vi "MT Calculate BER After Trigger (Fibonacci PN Sequence).vi"(0 "input bit stream":i8[](array[numeric]), 5 "PN sequence order (9)":i32=9, 7 "BER trigger threshold (0.1)":dbl=0.1 format="%.4f", 9 "confidence (0.95)":dbl=0.95 format="%.4f", 11 "error in (no error)":errorcluster, 13 "reset? (T)":bool=TRUE) -> (4 "BER":dbl format="%.4f", 6 "accumulated BER":dbl format="%.4f", 8 "trigger found?":bool, 10 "trigger found index (bits)":u32, 15 "error out":errorcluster)   [LabVIEW 2020, in "niDMT.lvlib"]
doc: "This polymorphic instance calculates the average BER against a Fibonacci PN sequence. The sequence must be the same as the PN sequence generated by the Fibonacci instance of the MT Generate Bits (poly) VI with a matching PN order."
uses:
  <vilib>/addons/Modulation/niDMT.lvlib
  <vilib>/addons/Modulation/niAMT.lvlib
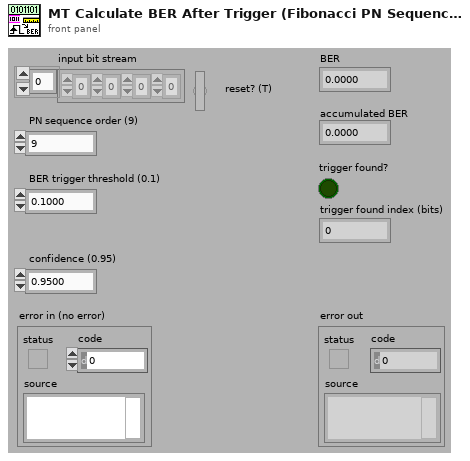
[diagram p1: front panel]
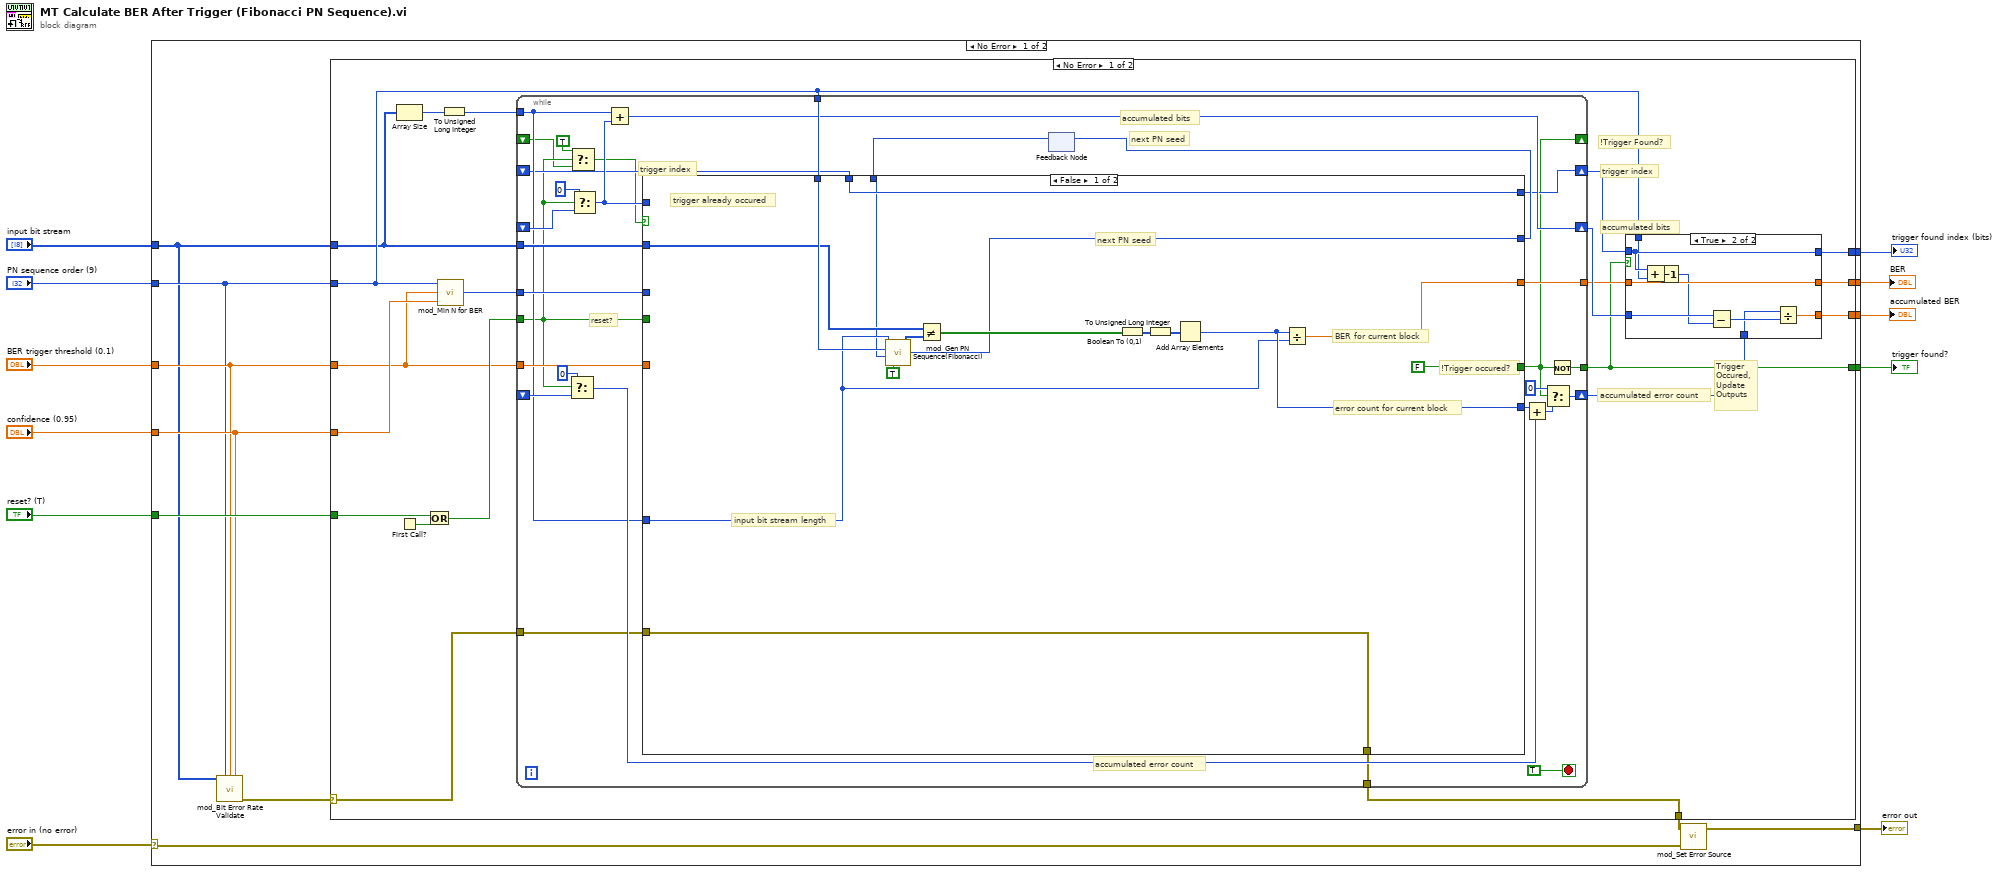
[diagram p0: block diagram]
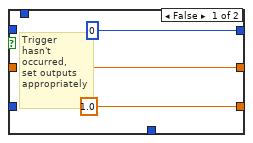
[diagram p2: hidden frame]
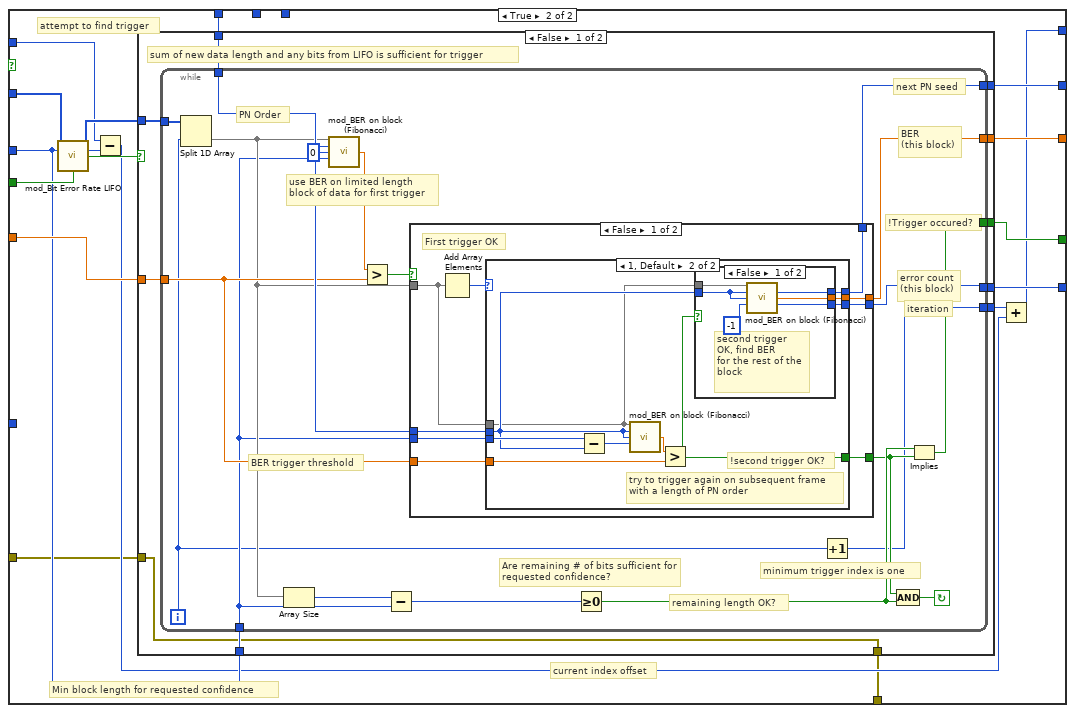
[diagram p3: hidden frame]
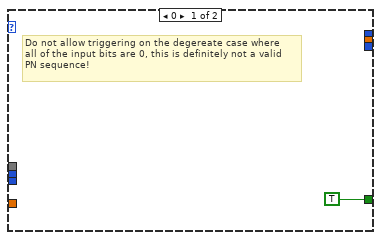
[diagram p4: hidden frame]
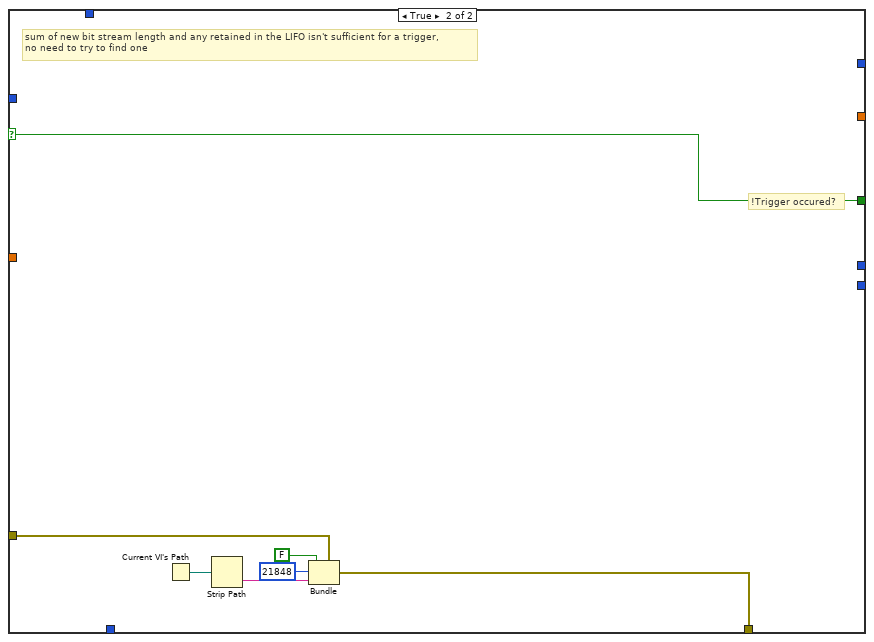
[diagram p7: hidden frame]
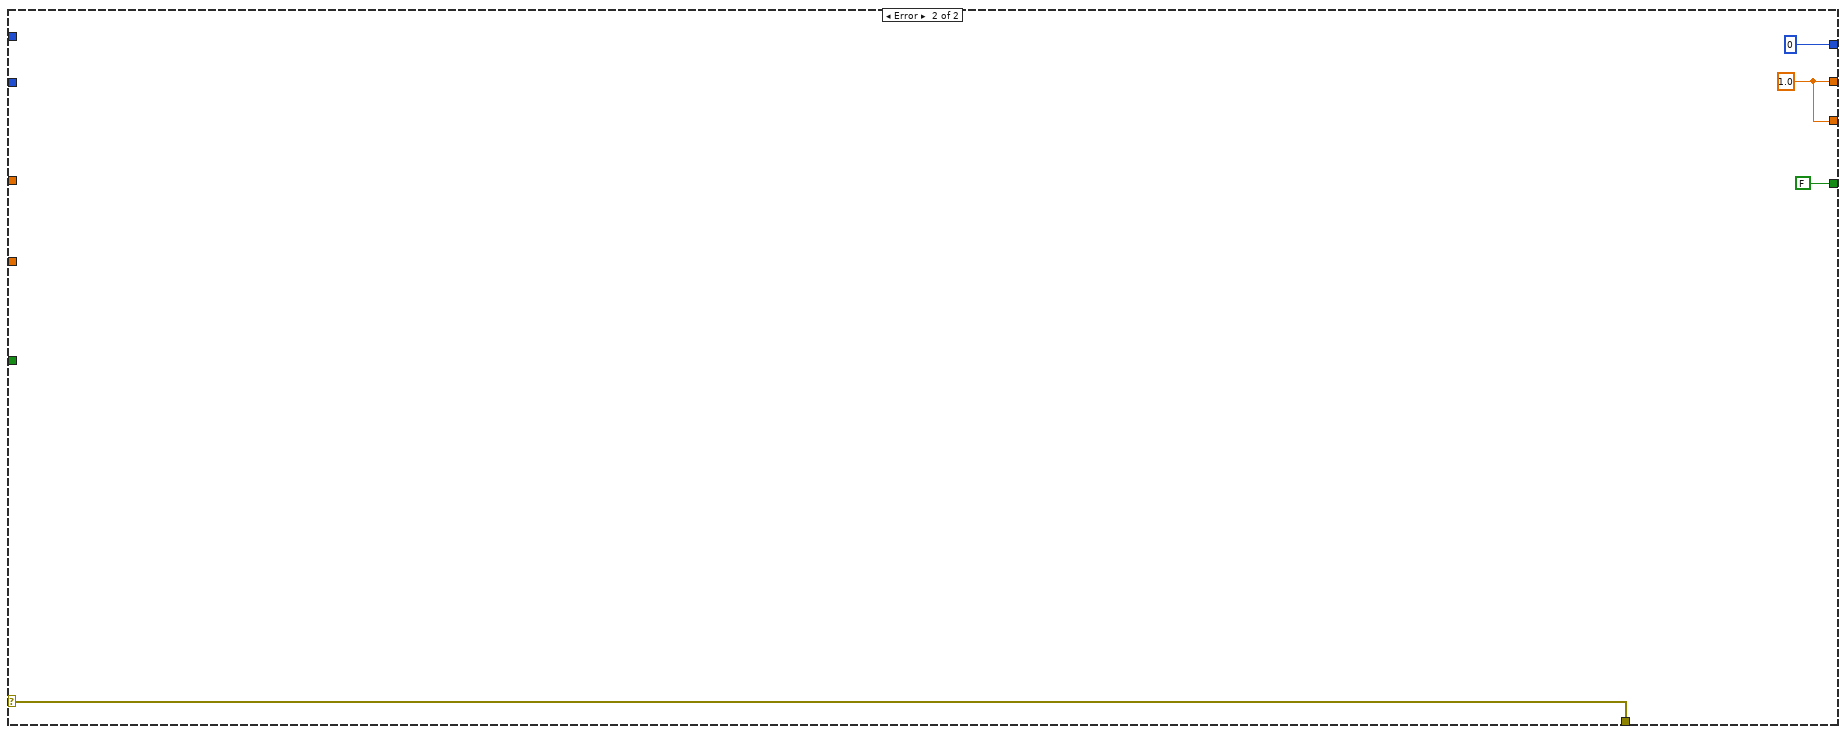
[diagram p8: hidden frame]
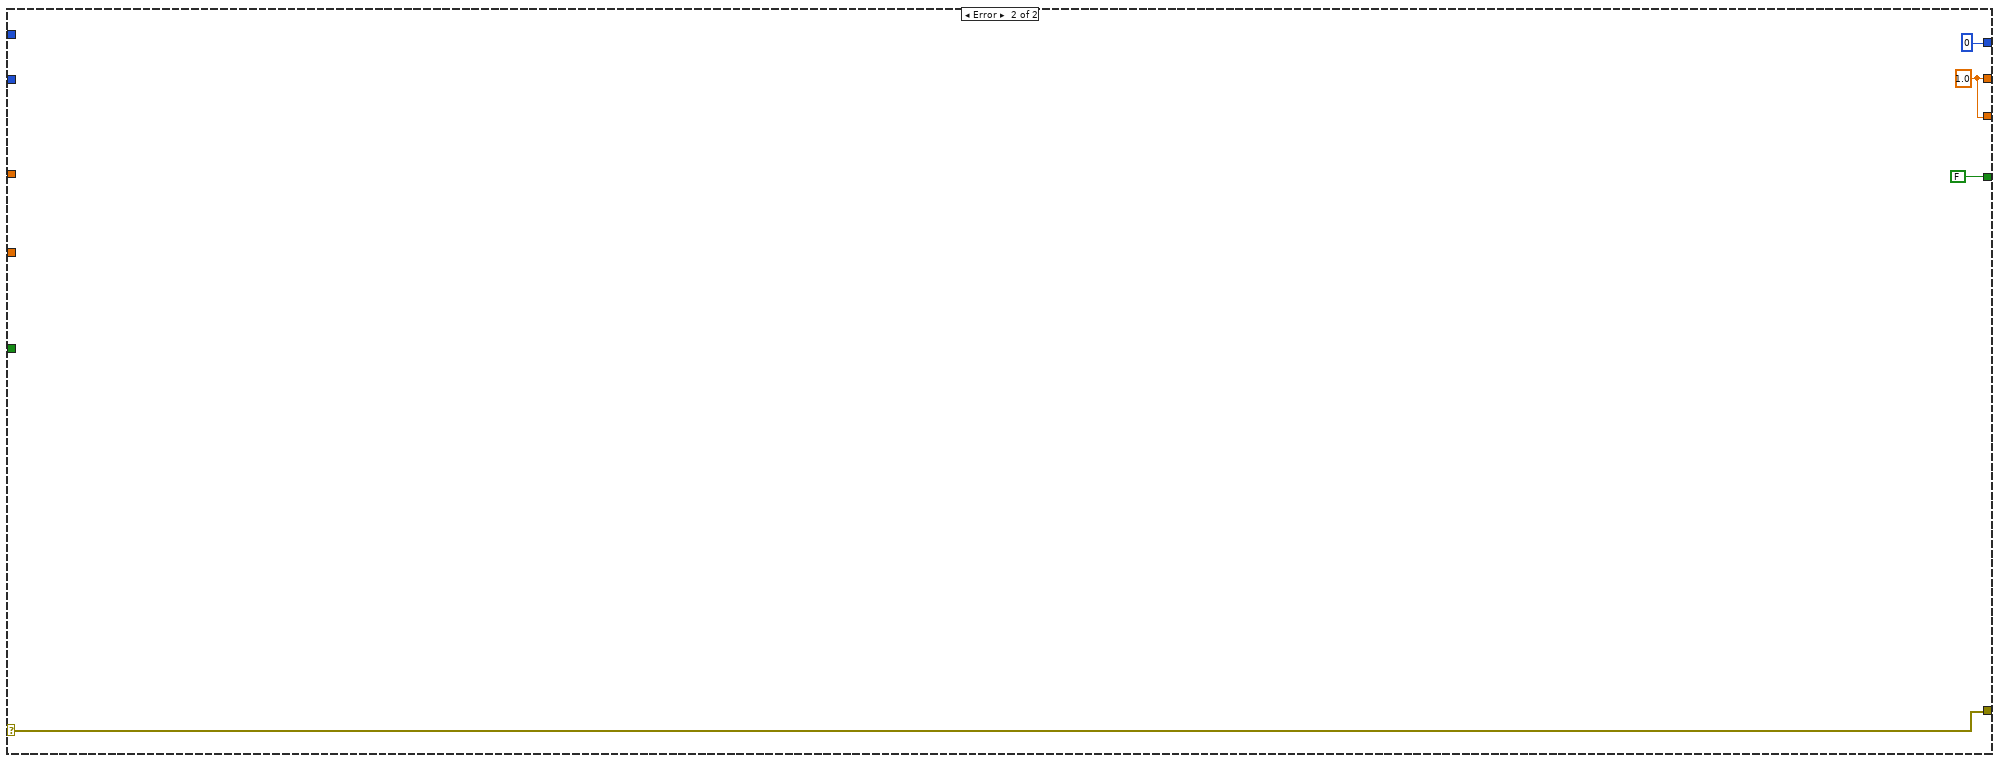
[diagram p9: hidden frame]
diagram:
  n1 = case shown="No Error" "error in (no error)" {
    selector: "error in (no error)" -> [w15 w189]
    tunnel: "reset? (T)" -> [w22 _]
    tunnel: "PN sequence order (9)" -> [w19 _]
    tunnel: "BER trigger threshold (0.1)" -> [w20 _]
    tunnel: "input bit stream" -> [w18 _]
    tunnel: [w24 w188] -> w8
    tunnel: "confidence (0.95)" -> [w21 _]
    tunnel: [w23 w189] -> w6
    tunnel: [w14 w188] -> w3
    tunnel: [w13 u32 0 ("t")] -> w2
    tunnel: [w12 FALSE] -> w1
    frame No Error {
      n2 = call <vilib>:"mod_Bit Error Rate Validate.vi"("Input Bit Stream"=w18, "PN Sequence Order (9)"=w19, "BER Sync Threshold (0.2)"=w20, "confidence (0.95)"=w21) -> ("error out"=w17:errorcluster)  [unwired: 1 in, 10 out]
      n3 = case shown="No Error" w17 {
        selector: w17 -> [w26 w185]
        tunnel: w19 -> [w30 _]
        tunnel: w20 -> [w31 _]
        tunnel: w18 -> [w28 _]
        tunnel: [w37 w184] -> w24
        tunnel: w21 -> [w32 _]
        tunnel: w22 -> [w40 _]
        tunnel: [w25 w185] -> w16
        tunnel: [w35 w184] -> w14
        tunnel: [w34 u32 0 ("t")] -> w13
        tunnel: [w33 FALSE] -> w12
        frame No Error {
          # "Trigger\nOccured,\nUpdate\nOutputs"
          # "!Trigger Found?"
          # "accumulated error count"
          # "trigger index"
          # "accumulated bits"
          n4 = Array Size(array=w28) -> (size(s)=w27:i32)
          n5 = First Call?() -> (First Call?: T/F=w42:bool)
          n6 = Or(x=w40, y=w42) -> (x .or. y?=w41:bool)
          n7 = call <vilib>:"mod_Min N for BER.vi"("confidence"=w32, "threshold"=w31, "PN sequence order"=w30) -> ("min N"=w29:i32)
          n8 = To Unsigned Long Integer(number=w27) -> (unsigned 32bit integer=w36:u32)
          n9 = while {
            shift-right: [w65] -> w39
            shift-left: _ -> [w62]
            tunnel: w41 -> [w61]
            tunnel: w28 -> [w77]
            tunnel: w29 -> [w84]
            tunnel: w30 -> [w83]
            tunnel: w31 -> [w81]
            shift-right: [w67] -> w44
            shift-left: _ -> [w78]
            tunnel: [w80] -> w38
            shift-right: [w74] -> w43
            shift-left: _ -> [w70]
            tunnel: w36 -> [w66]
            tunnel: [w64] -> w33
            shift-right: [w63] -> _
            shift-left: _ -> [w60]
            tunnel: w26 -> [w57]
            tunnel: [w56] -> w25
            stop <- TRUE stop-if-true
            # "accumulated error count"
            # "accumulated bits"
            # "next PN seed"
            # "reset?"
            # "trigger index"
            n10 = Select(t=u32 0, s=w61, f=w70) -> (s? t:f=w69:u32)
            n11 = Select(t=TRUE, s=w61, f=w60) -> (s? t:f=w58:bool)
            n12 = Select(t=u32 0, s=w61, f=w78) -> (s? t:f=w68:u32)
            n13 = Add(x=w66, y=w68) -> (x+y=w67:u32)
            n14 = feedback #1() -> (w72:u32)  [unwired: 1 out]
            n15 = case shown="False" w58 {
              tunnel: w77 -> [w91 w117]
              tunnel: w84 -> [_ w113]
              tunnel: w61 -> [_ w118]
              tunnel: w83 -> [w98 w116]
              tunnel: [w86 w115] -> w82
              tunnel: w81 -> [_ w114]
              tunnel: [w96 w112] -> w80
              tunnel: w68 -> [_ w105]
              tunnel: w62 -> [w97 _]
              tunnel: [w97 w103] -> w65
              tunnel: [FALSE w110] -> w63
              tunnel: [w99 w109] -> w76
              tunnel: w72 -> [w87 _]
              tunnel: w66 -> [w88 _]
              tunnel: w57 -> [w89 w102]
              tunnel: [w89 w101] -> w56
              frame False {
                # "input bit stream length"
                # "!Trigger occured?"
                # "BER for current block"
                # "error count for current block"
                # "trigger already occured"
                # "next PN seed"
                n16 = call <vilib>:"mod_Gen PN Sequence(Fibonacci).vi"("total bits (128)"=w88, "PN sequence order"=w98, "seed in (0xD6BF7DF2)"=w87, "reset? (T)"=TRUE ("Reset? (T)")) -> ("output bit stream"=w95:i8[], "seed out"=w86:i32)  [unwired: 1 in, 1 out]
                n17 = Not Equal?(x=w91, y=w95) -> (x != y?=w92:bool[])
                n18 = Boolean To (0,1)(Boolean=w92) -> (0, 1=w93:i16[])
                n19 = To Unsigned Long Integer(number=w93) -> (unsigned 32bit integer=w90:u32[])
                n20 = Add Array Elements(numeric array=w90) -> (sum=w99:u32)
                n21 = Divide(x=w99, y=w88) -> (x/y=w96:dbl)
              }
              frame True {
                # "Min block length for requested confidence"
                # "current index offset"
                # "attempt to find trigger"
                n22 = call <vilib>:"mod_Bit Error Rate LIFO.vi"("input bit stream"=w117, "max buffer length"=w113, "reset"=w118) -> ("output bit stream"=w111:i8[], "Old Buffer Length (Prior to New Bits)"=w106:i32, "Updated Buffer Length less \nthan max length"=w108:bool)  [unwired: 10 out]
                n23 = Subtract(x=w105, y=w106) -> (x-y=w104:u32)
                n24 = case shown="False" w108 {
                  selector: w108 -> [_ w181]
                  tunnel: w116 -> [w128 _]
                  tunnel: [w127 _] -> w115
                  tunnel: w114 -> [w126 _]
                  tunnel: w113 -> [w125 _]
                  tunnel: [w124 _] -> w112
                  tunnel: w111 -> [w123 _]
                  tunnel: [w122 w181] -> w110
                  tunnel: [w121 _] -> w109
                  tunnel: [w120 _] -> w107
                  tunnel: w102 -> [w119 w179]
                  tunnel: [w119 w175] -> w101
                  frame False {
                    # "sum of new data length and any bits from LIFO is sufficient for trigger"
                    n25 = while {
                      tunnel: w128 -> [w141]
                      tunnel: w123 -> [w147]
                      tunnel: [w143] -> w127
                      tunnel: w126 -> [w138]
                      tunnel: w125 -> [w132]
                      tunnel: [w145] -> w124
                      tunnel: [w133] -> w122
                      tunnel: [w129] -> w120
                      tunnel: [w144] -> w121
                      i -> [w130]
                      stop <- w142 continue-if-true
                      # "minimum trigger index is one"
                      # "remaining length OK?"
                      # "BER\n(this block)"
                      # "error count\n(this block)"
                      # "iteration"
                      # "Are remaining # of bits sufficient for requested confidence?"
                      # "BER trigger threshold"
                      # "!Trigger occured?"
                      # "PN Order"
                      # "use BER on limited length\nblock of data for first trigger"
                      # "next PN seed"
                      n26 = Split 1D Array(array=w147, index=w130) -> (second subarray=w136:i8[])  [unwired: 1 out]
                      n27 = Array Size(array=w136) -> (size(s)=w137:i32)
                      n28 = call <vilib>:"mod_BER on block (Fibonacci).vi"("bit stream in"=w136, "expected PN sequence order"=w141, "starting index"=0, "length (0 or negative = entire block)"=w132) -> ("BER"=w139:dbl)  [unwired: 11 out]
                      n29 = Greater?(x=w139, y=w138) -> (0:w140:bool)
                      n30 = Subtract(x=w137, y=w132) -> (x-y=w146:i32)
                      n31 = case shown="False" w140 {
                        selector: w140 -> [_ w174]
                        tunnel: w136 -> [w149 _]
                        tunnel: [w155 _] -> w145
                        tunnel: w141 -> [w150 _]
                        tunnel: [w154 _] -> w144
                        tunnel: [w156 _] -> w143
                        tunnel: [w152 w174] -> w134
                        tunnel: w138 -> [w153 _]
                        tunnel: w132 -> [w151 _]
                        frame False {
                          # "First trigger OK"
                          n32 = Add Array Elements(numeric array=w149) -> (sum=w148:i8)
                          n33 = case shown="1, Default" w148 {
                            tunnel: [_ w167] -> w156
                            tunnel: [_ w166] -> w155
                            tunnel: [_ w165] -> w154
                            tunnel: w153 -> [_ w163]
                            tunnel: [TRUE w161] -> w152
                            tunnel: w151 -> [_ w160]
                            tunnel: w150 -> [_ w159]
                            tunnel: w149 -> [_ w158]
                            frame 0 {
                              # "Do not allow triggering on the degereate case where\nall of the input bits are 0, this is definitely not a valid\nPN sequence!"
                            }
                            frame 1, Default {
                              # "!second trigger OK?"
                              # "try to trigger again on subsequent frame\nwith a length of PN order"
                              n34 = Subtract(x=w160, y=w159) -> (x-y=w162:i32)
                              n35 = call <vilib>:"mod_BER on block (Fibonacci).vi"("bit stream in"=w158, "expected PN sequence order"=w159, "starting index"=w159, "length (0 or negative = entire block)"=w162) -> ("BER"=w164:dbl)  [unwired: 11 out]
                              n36 = Greater?(x=w164, y=w163) -> (0:w161:bool)
                              n37 = case shown="False" w161 {
                                tunnel: [w173 _] -> w167
                                tunnel: [w172 _] -> w166
                                tunnel: [w171 _] -> w165
                                tunnel: w158 -> [w170 _]
                                tunnel: w159 -> [w168 _]
                                frame False {
                                # "second trigger\nOK, find BER\nfor the rest of the\nblock"
                                n38 = call <vilib>:"mod_BER on block (Fibonacci).vi"("bit stream in"=w170, "expected PN sequence order"=w168, "starting index"=w168, "length (0 or negative = entire block)"=-1 ("length")) -> ("next seed"=w173:u32, "BER"=w172:dbl, "number of errors"=w171:u32)  [unwired: 9 out]
                                }
                                frame True {
                                }
                              }
                            }
                          }
                        }
                        frame True {
                        }
                      }
                      n39 = Greater Or Equal To 0?(x=w146) -> (x >= 0?=w135:bool)
                      n40 = Increment(x=w130) -> (x+1=w129:i32)
                      n41 = Compound Arithmetic op=AND(w134, w135) -> (w142:bool)
                      n42 = Implies(1:w134, 2:w135) -> (0:w133:bool)
                    }
                  }
                  frame True {
                    # "!Trigger occured?"
                    # "sum of new bit stream length and any retained in the LIFO isn't sufficient for a trigger,\nno need to try to find one"
                    n43 = Current VI's Path() -> (path=w180:path)
                    n44 = Strip Path(path=w180) -> (name=w177:string)  [unwired: 1 out]
                    n45 = Bundle(cluster=w179, "status"=FALSE, "code"=21848, "source"=w177) -> (w175:errorcluster)
                  }
                }
                n46 = Add(x=w107, y=w104) -> (x+y=w103:u32)
              }
            }
            n47 = feedback-in #1(w82) -> ()
            n48 = Add(x=w76, y=w69) -> (x+y=w75:u32)
            n49 = Select(t=u32 0, s=w63, f=w75) -> (s? t:f=w74:u32)
            n50 = Not(x=w63) -> (.not. x?=w64:bool)
          }
          n51 = case shown="True" w33 {
            tunnel: w44 -> [_ w52]
            tunnel: w43 -> [_ w51]
            tunnel: [w46 w55] -> w35
            tunnel: w39 -> [_ w50]
            tunnel: w38 -> [_ w54]
            tunnel: [w46 w54] -> w37
            tunnel: [u32 0 ("t") w50] -> w34
            tunnel: w30 -> [_ w49]
            frame False {
              w46 = 1.0 ("f")
              # "Trigger\nhasn't \noccurred,\nset outputs\nappropriately"
            }
            frame True {
              n52 = Add(x=w50, y=w49) -> (x+y=w48:u32)
              n53 = Decrement(x=w48) -> (x-1=w47:u32)
              n54 = Subtract(x=w52, y=w47) -> (x-y=w53:u32)
              n55 = Divide(x=w51, y=w53) -> (x/y=w55:dbl)
            }
          }
        }
        frame Error {
          w184 = 1.0
        }
      }
      n56 = call <vilib>:"mod_Set Error Source.vi"("initial error in (no error)"=w15, "final error in (no error)"=w16) -> ("error out"=w23:errorcluster)  [unwired: 3 out]
    }
    frame Error {
      w188 = 1.0
    }
  }
  "BER" <- w8
  "error out" <- w6
  "accumulated BER" <- w3
  "trigger found index (bits)" <- w2
  "trigger found?" <- w1
